vi "Destroy.vi"(8 "error in (no error)":errorcluster, 11 "reference in":refnum<class "BaseObject.lvclass">) -> (0 "error out":errorcluster, 3 "reference out":refnum<class "BaseObject.lvclass">)   [LabVIEW 2014, in "BaseClasses.lvlib" / "BaseObject.lvclass"]
uses:
  BaseObject.lvclass
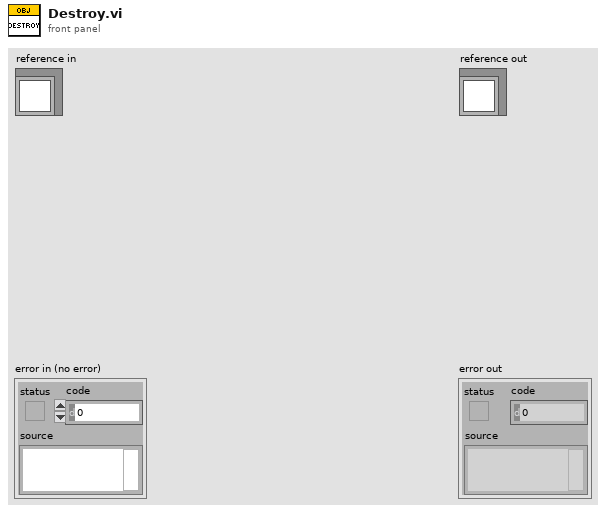
[diagram p1: front panel]
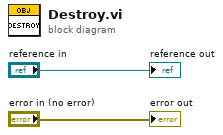
[diagram p0: block diagram]
diagram:
  "error out" <- "error in (no error)"
  "reference out" <- "reference in"
